vi "Init.vi"(6 "Position":T1, 7 "Round":u32, 9 "Team in":refnum<class "Team.lvclass">, 10 "Board Size":i32, 11 "Square in":refnum<class "Square.lvclass">) -> (1 "Team out":refnum<class "Team.lvclass">, 3 "Square out":refnum<class "Square.lvclass">)   [LabVIEW 2020, in "SquareBattle.lvlib" / "Square.lvclass"]
uses:
  Square.lvclass
  Team/Team.lvclass
  Position.ctl
  Team/Team.lvclass/Team.ctl
  Square.lvclass/Square.ctl
  Team Stats.ctl
  SquareBattle.lvlib
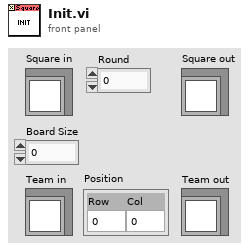
[diagram p1: front panel]
types:
  T1 = typedef "SquareBattle.lvlib/Position.ctl" = cluster{"Row":i32, "Col":i32}
  T2 = typedef "SquareBattle.lvlib/Team Stats.ctl" = cluster{"Active":i32, "Generated":i32, "Kills":i32, "Eliminated":i32, "Collided":i32}
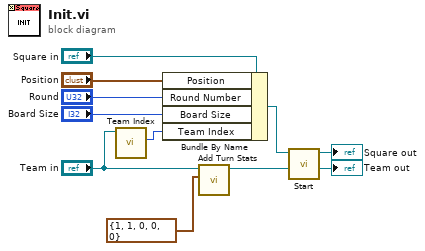
[diagram p0: block diagram]
diagram:
  n1 = call "Team Index.vi"("Team"="Team in") -> ("Team Index"=w9:i32)  [unwired: 10 in]
  n2 = Bundle By Name(cluster="Square in", "Position"="Position", "Round Number"="Round", "Board Size"="Board Size", "Team Index"=w9) -> (w8:refnum<class "Square.lvclass">)
  n3 = call "Add Turn Stats.vi"("Team Stats"=T2 {"Active"=1, "Generated"=1, "Kills"=0, "Eliminated"=0, "Collided"=0}, "Team in"="Team in") -> ("Team out"=w1:refnum<class "Team.lvclass">)  [unwired: 9 in]
  n4 = call-dynamic "Start.vi"("Team In"=w1, "Square in"=w8) -> ("Team"=→"Team out":refnum<class "Team.lvclass">, "Square out"=→"Square out":refnum<class "Square.lvclass">)  [unwired: 8 in]
